vi "AIMove_MinMax.vi"(1 "Player":i32, 2 "input board":i32[][](array[numeric])) -> (0 "column":i32)   [LabVIEW 2025]
uses:
  <vilib>/MakerHub/Toolbox/LMH-Toolbox.lvlib
panel:
  out "error out":errorcluster
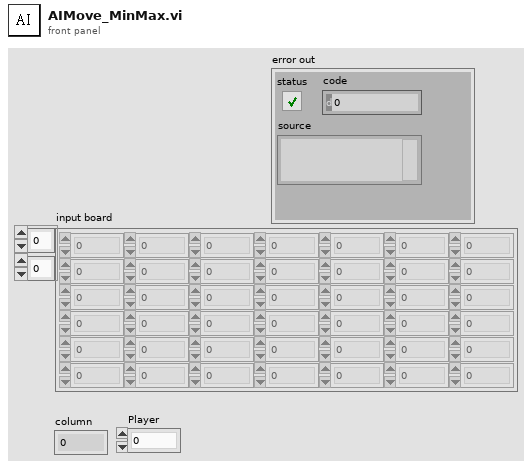
[diagram p1: front panel]
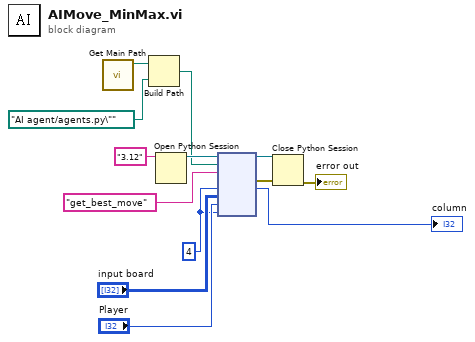
[diagram p0: block diagram]
diagram:
  w4 = 4
  n1 = call <vilib>:"Get Main Path.vi"() -> ("Main Dir"=w2:path)  [unwired: 9 in, 2 out]
  n2 = Build Path(base path=w2, name or relative path=path "AI agent/agents.py\"" ("module path")) -> (appended path=w1:path)
  n3 = Open Python Session(python version="3.12" ("Python version")) -> (session out=w12:refnum<k35>)  [unwired: 2 in, 1 out]
  n4 = node(w12, w1, "get_best_move" ("function name"), w4, "input board", "Player", w4) -> (w10:refnum<k35>, w9:errorcluster, →"column":i32)  [unwired: 4 in, 2 out]
  n5 = Close Python Session(session in=w10, error in=w9) -> (11:→"error out":errorcluster)
